vi "TestCloneAPI.vi"() -> ()   [LabVIEW 2018, in "SpecAnModule.lvlib"]
uses:
  SpecAnModule.lvlib
  TestInfo.ctl
  <userlib>/NIST/ModuleAdminLib/CloneRegistration/CloneRegistration.lvclass
  <userlib>/NIST/ModuleAdminLib/ModuleAdmin/ModuleAdmin.lvclass/ModuleAdmin.ctl
  <userlib>/NIST/ModuleAdminLib/ModuleAdmin/ModuleAdmin.lvclass
  PublicAPI/Arguments/Broadcasts/clDidInit.ctl
  PublicAPI/Arguments/Requests/clStopArgument.ctl
  SpecAnPlugins/SpecAnBaseClass/Typedefs/Waveform(s).ctl
  <userlib>/NIST/ModuleAdminLib/ModuleAdmin/Accessors/Read CloneRegRef.vi
  <userlib>/NIST/ModuleAdminLib/ModuleAdmin/Accessors/Write CloneRegRef.vi
  SpecAnPlugins/SpecAnBaseClass/SpecAnBase.lvclass
panel:
  out "Actual Points":i32[](array[numeric])
  out "Waveform Graph":T1(graph)
  in  "option string":string="Simulate=1,RangeCheck=1,QueryInstrStatus=0,Cache=1"
  in  "reset device (Yes)":bool=TRUE
  in  "id query (Yes)":bool=TRUE
  in  "btnAcqMode":bool
  out "TraceNames":string[](array[string])
  in  "btnInitiate":bool
  in  "btnGetTraceName":bool
  in  "btnConfigure":bool
  in  "btnAbortDevice":bool
  in  "btnCloseDevice":bool
  in  "btnInitDevice":bool
  in  "btnClear":bool
  in  "btnPref":bool
  in  "Show Panel":bool=TRUE
  in  "Plugin Type":u16(ring) items=["IVI Spectrum Analyzer"]
  in  "btnLoadPlugin":bool
  out "Path":path
  in  "btnRequestINIPath":bool
  in  "btnRemove":bool
  out "Status Log":string
  out "Active Modules (Array)":string[](array[string])
  in  "btnAdd":bool
  in  "btnStop":bool
  in  "Select Module":i32(ring)=-1 caption="Select Module to send Request" items=["All"=-1, "4140002"=4140002]
  # "Hidden"
  # "Visible"
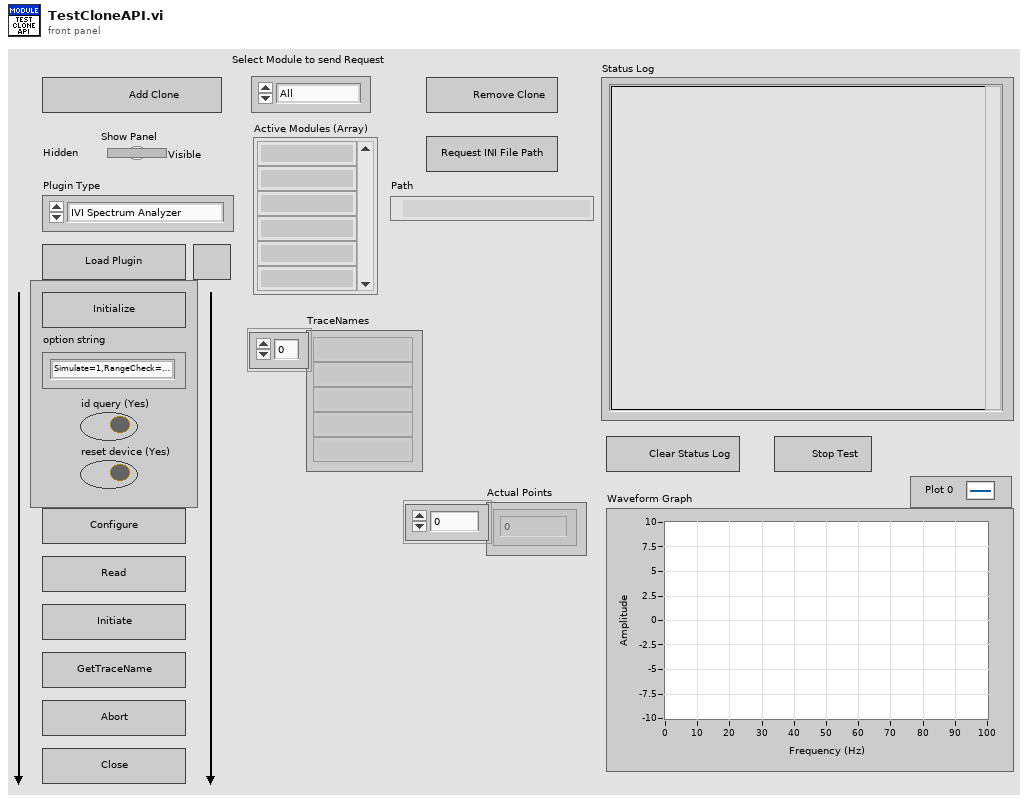
[diagram p1: front panel]
types:
  T1 = cluster{"Start Frequency (Hz)":dbl, "Delta Frequency(Hz)":dbl, "Amplitude":dbl[][]}
  T2 = typedef "SpecAnModule.lvlib/TestInfo.ctl" = cluster{"PluginIniFilePaths":path[]}
  T3 = cluster{"Status Log":refnum<vi>, "btnAdd":refnum<vi>, "btnStop":refnum<vi>, "Show Panel":refnum<vi>, "btnClear":refnum<vi>}
  T4 = typedef "SpecAnModule.lvlib/clBroadcastEvents.ctl" = cluster{"DidInit":refnum<user-event>, "StatusUpdate":refnum<user-event>, "ErrorReport":refnum<user-event>, "DidStop":refnum<user-event>, "PathToINI":refnum<user-event>, "TraceName":refnum<user-event>, "Reload Configuration File(s)":refnum<user-event>, "Measurements":refnum<user-event>}
  T5 = enum8{"Enabled", "Disabled", "Disabled and Grayed Out"}
  T6 = typedef "SpecAnModule.lvlib/clDidInit.ctl" = cluster{"Init?":bool, "ModuleAdmin":refnum<class "ModuleAdmin.lvclass">}
  T7 = typedef "SpecAnModule.lvlib/clStopArgument.ctl" = cluster{"Exit via Stop Module Req?":bool, "Wait for Module to stop?":bool, "ModuleAdmin":refnum<class "ModuleAdmin.lvclass">}
  T8 = typedef "SpecAnPlugins.lvlib/SpecAnBase.lvclass/Waveform(s).ctl" = cluster{"Actual Points":i32[], "Waveform Data":cluster{"Start Frequency (Hz)":dbl, "Delta Frequency(Hz)":dbl, "Amplitude":dbl[][]}}
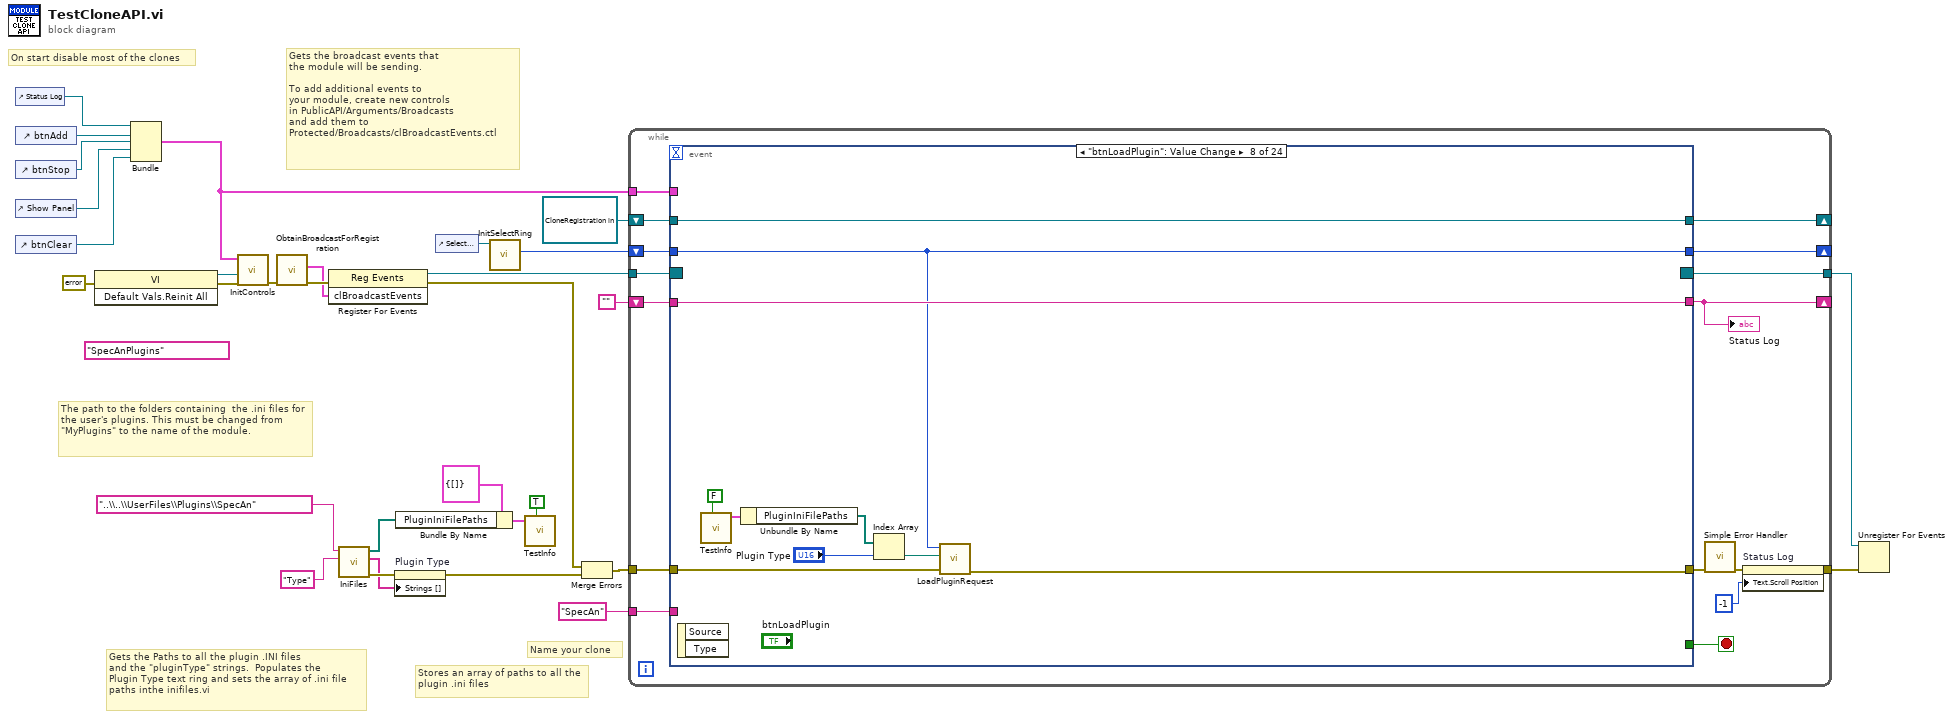
[diagram p0: block diagram]
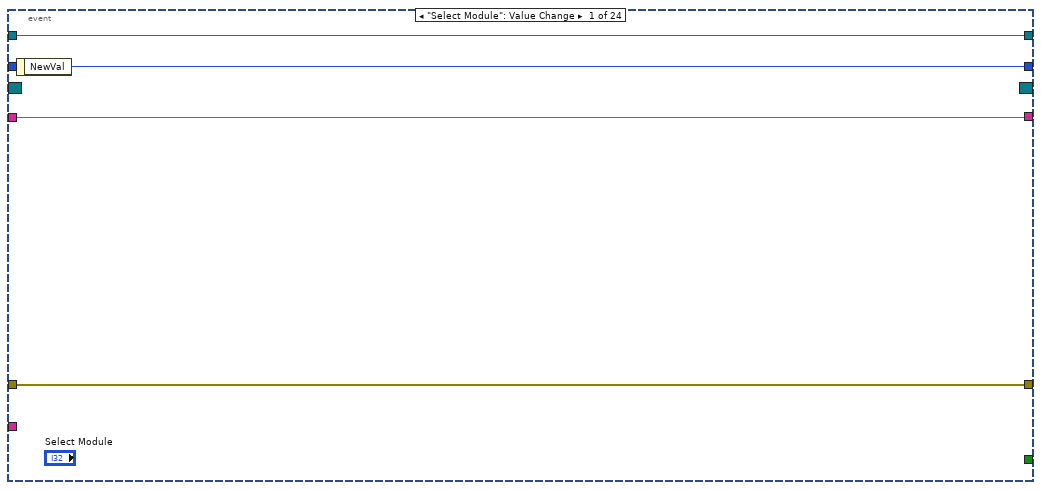
[diagram p2: hidden frame]
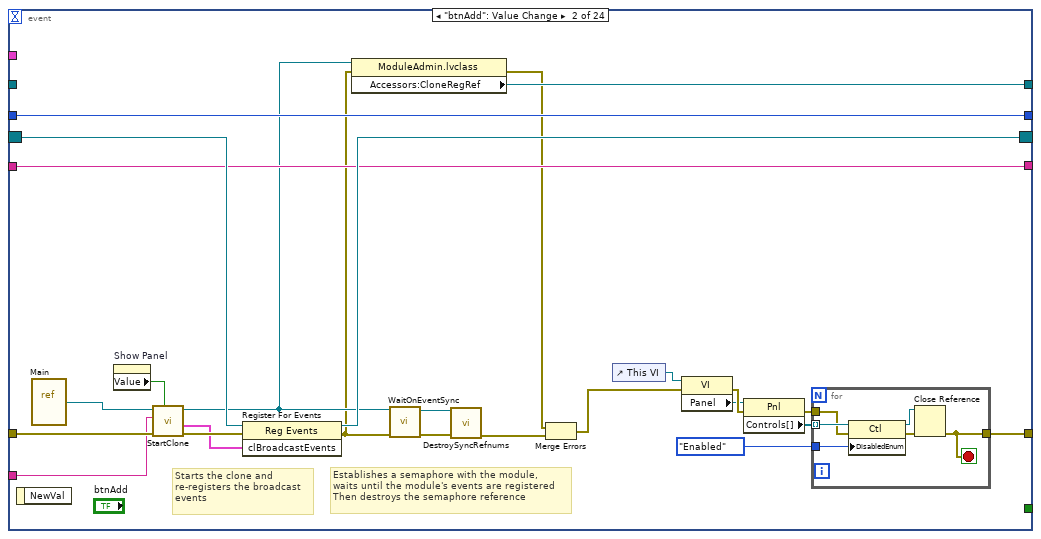
[diagram p3: hidden frame]
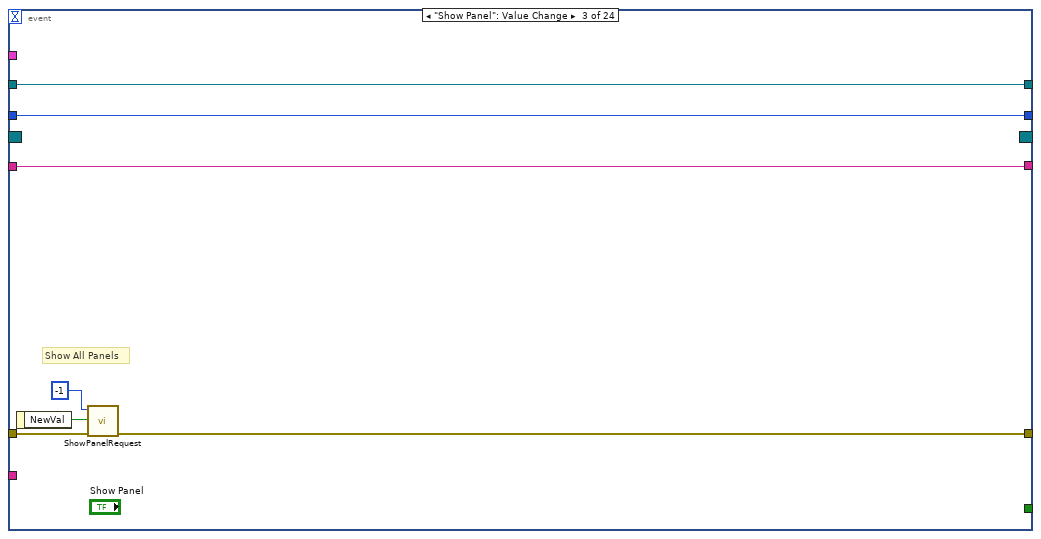
[diagram p4: hidden frame]
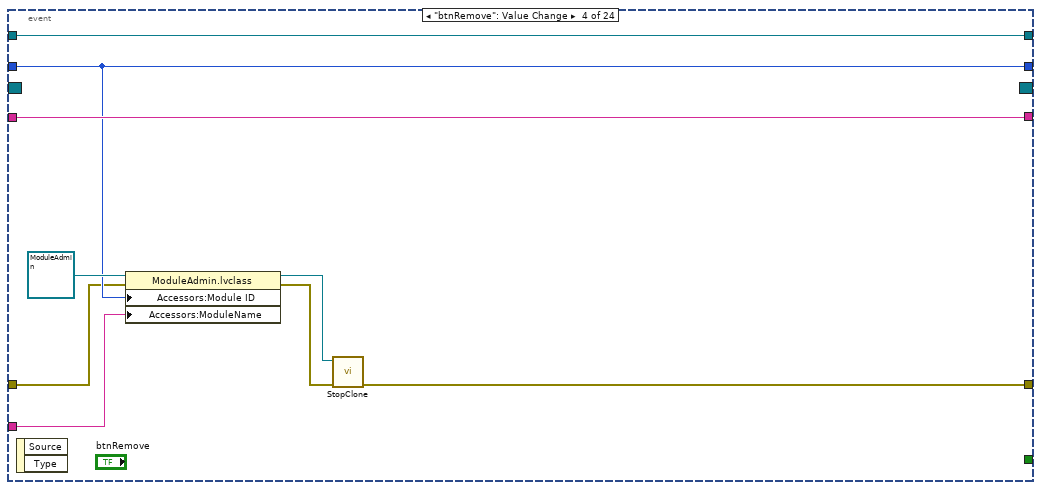
[diagram p5: hidden frame]
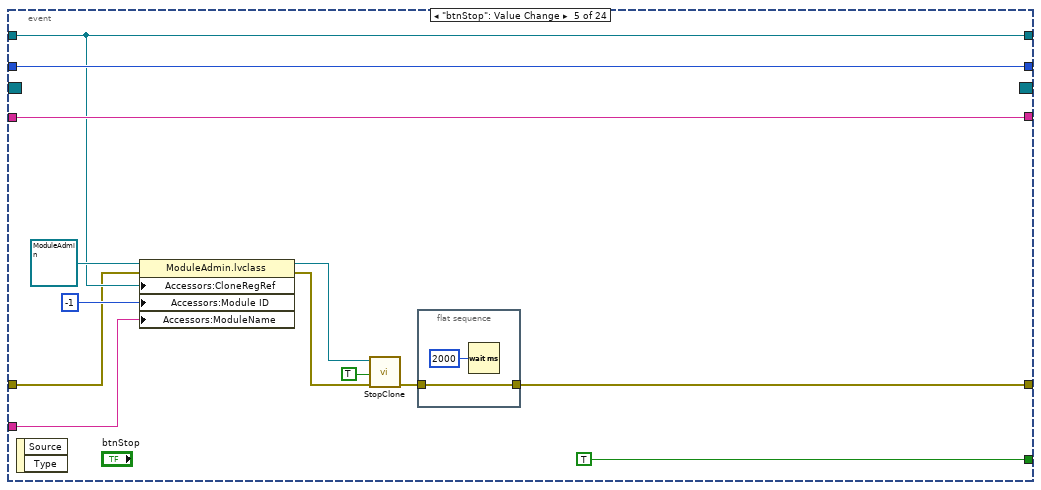
[diagram p6: hidden frame]
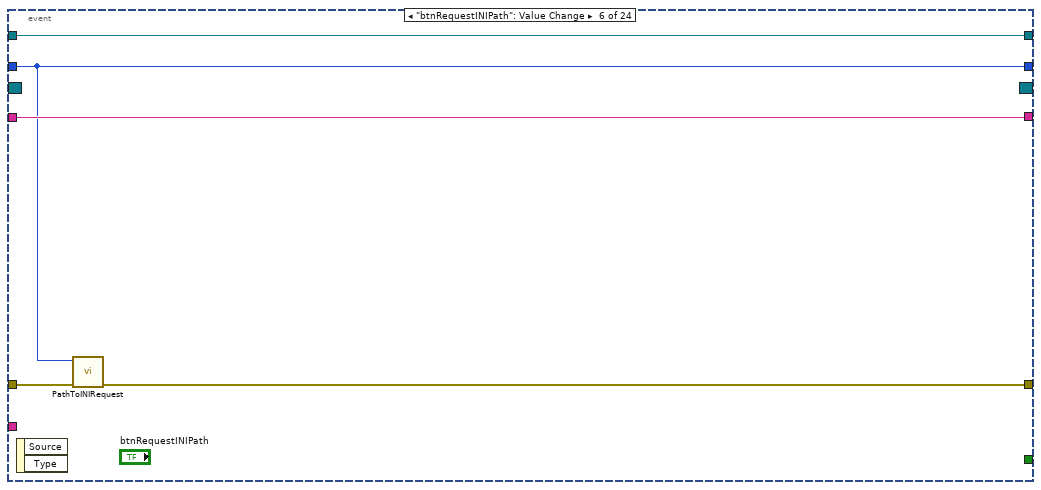
[diagram p7: hidden frame]
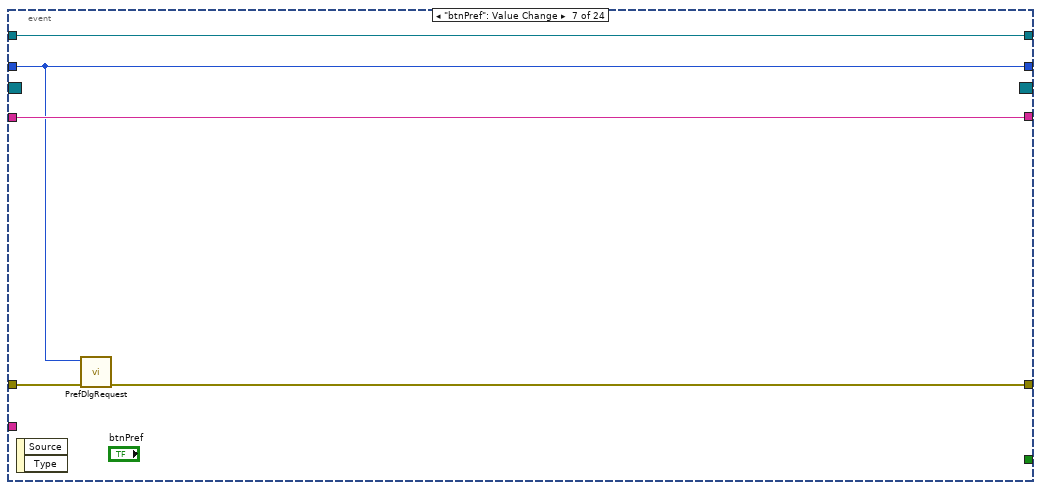
[diagram p8: hidden frame]
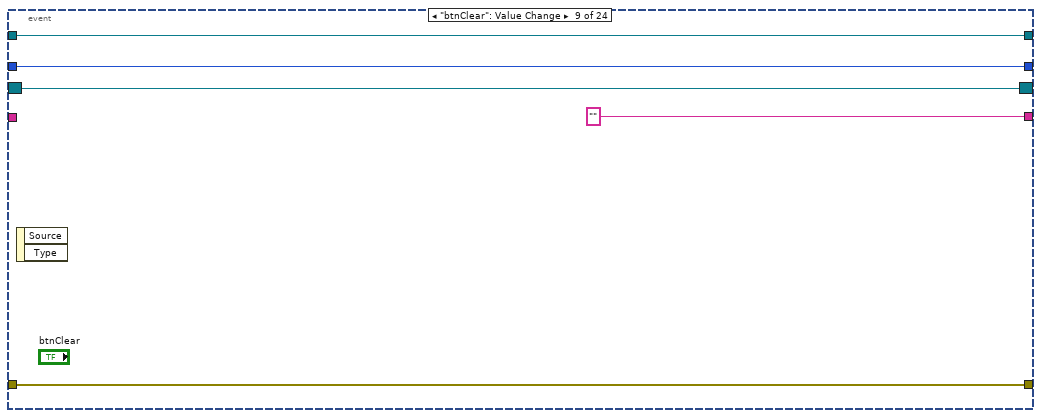
[diagram p9: hidden frame]
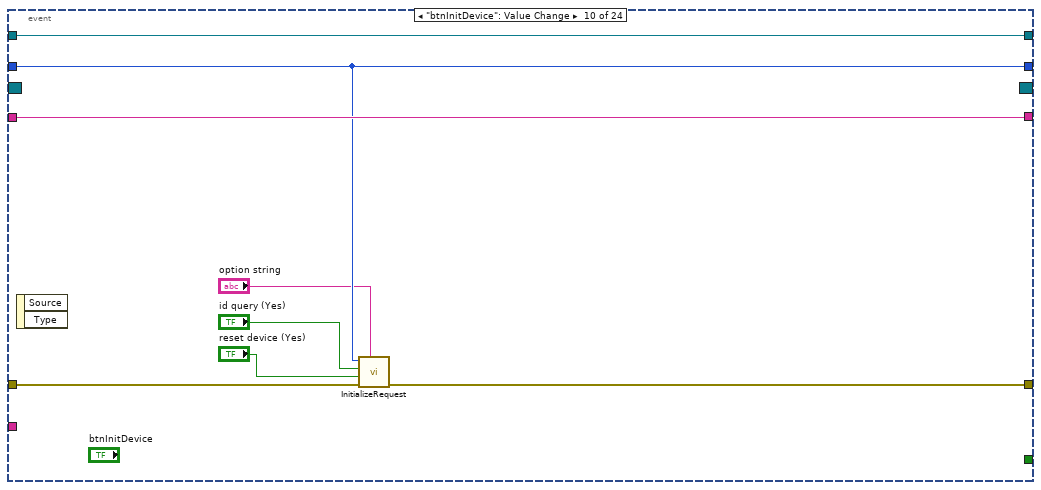
[diagram p10: hidden frame]
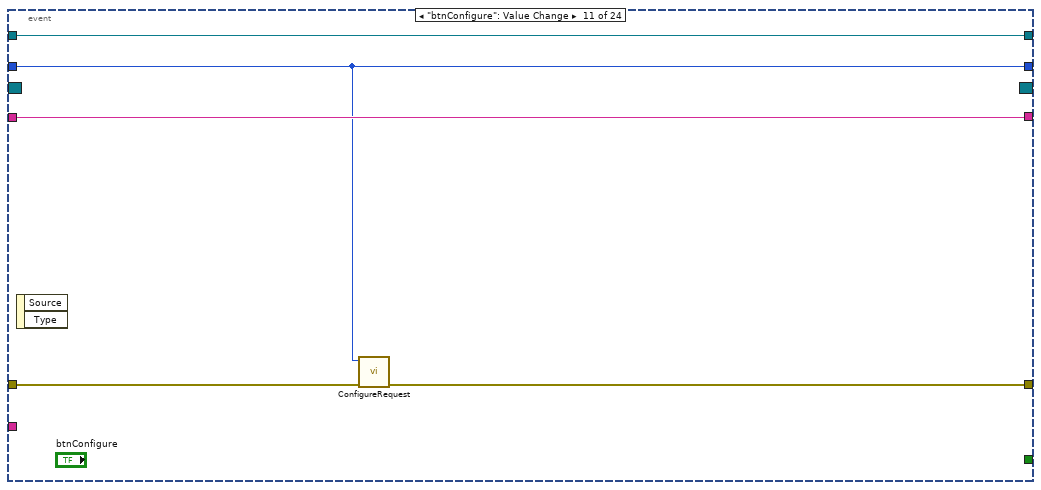
[diagram p11: hidden frame]
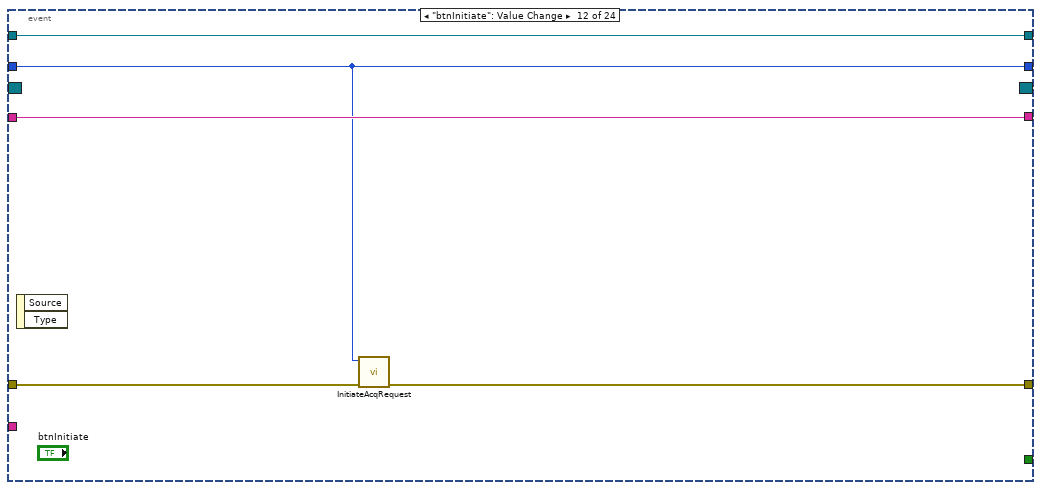
[diagram p12: hidden frame]
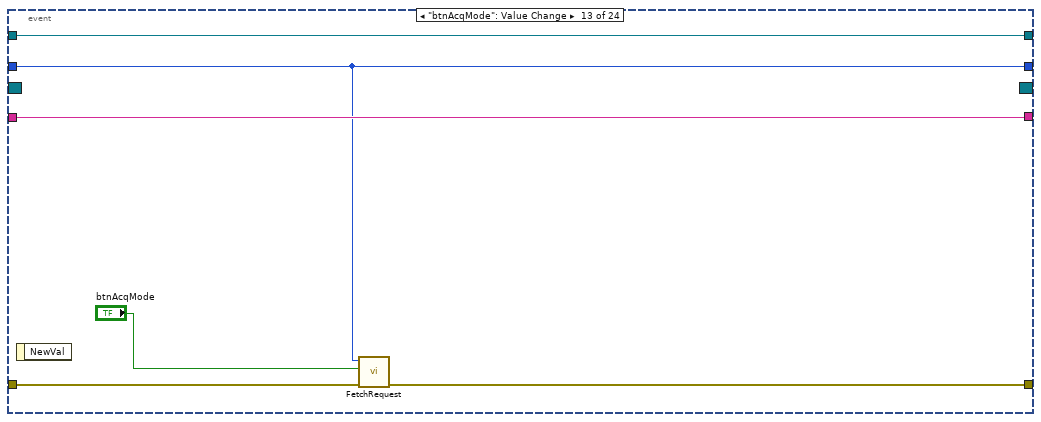
[diagram p13: hidden frame]
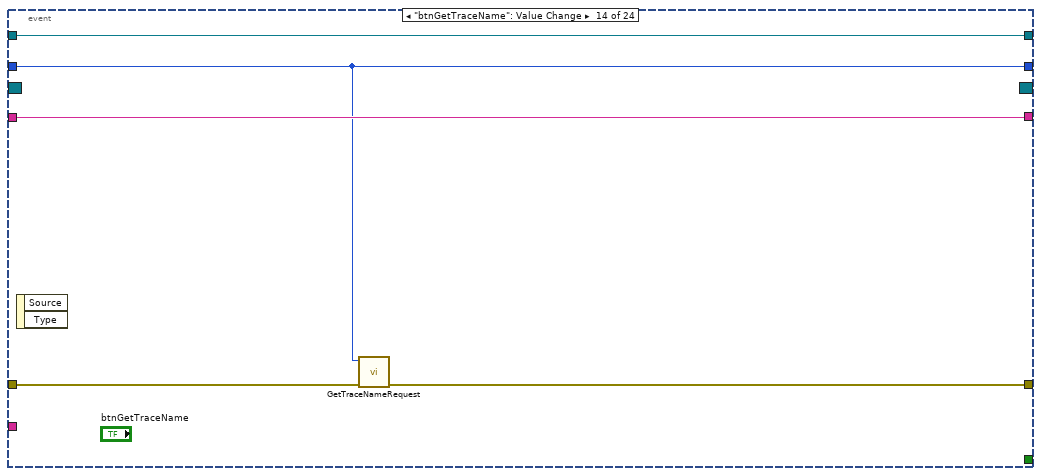
[diagram p14: hidden frame]
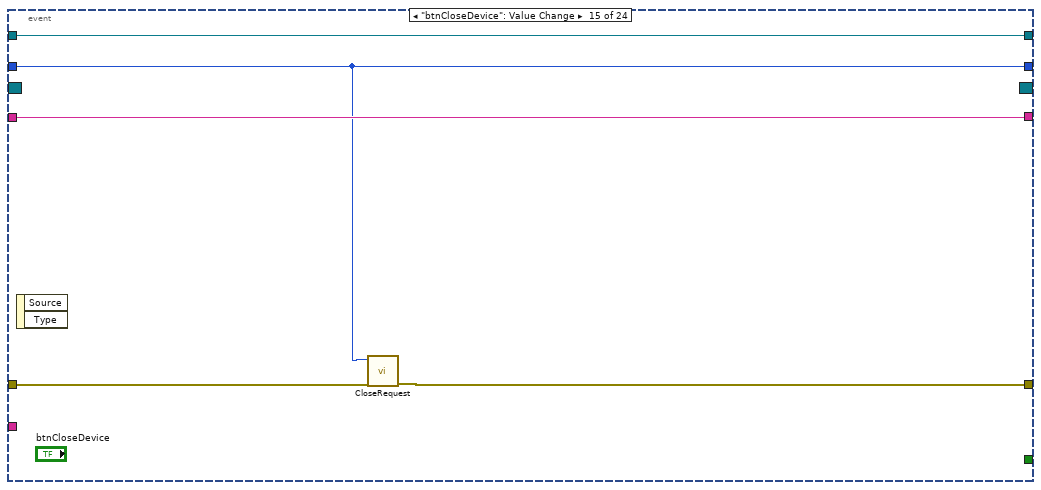
[diagram p15: hidden frame]
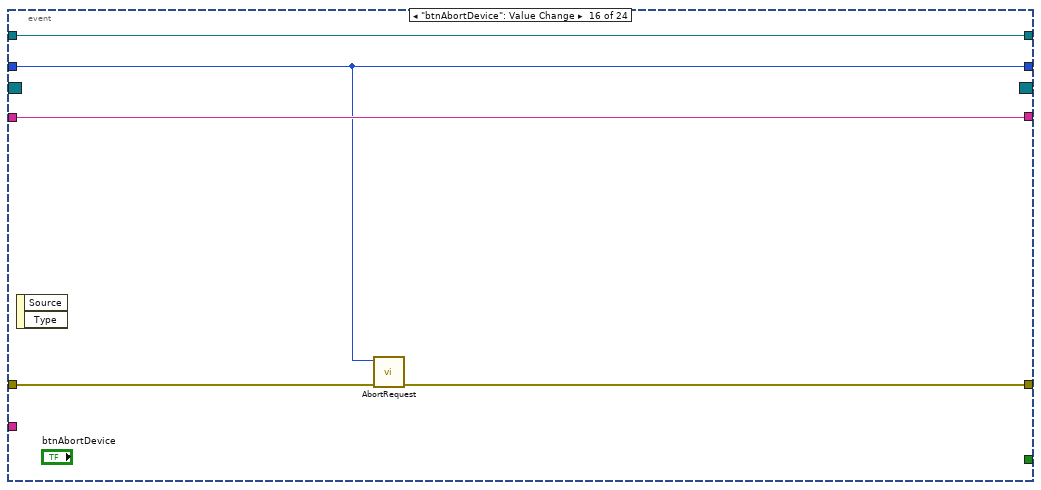
[diagram p16: hidden frame]
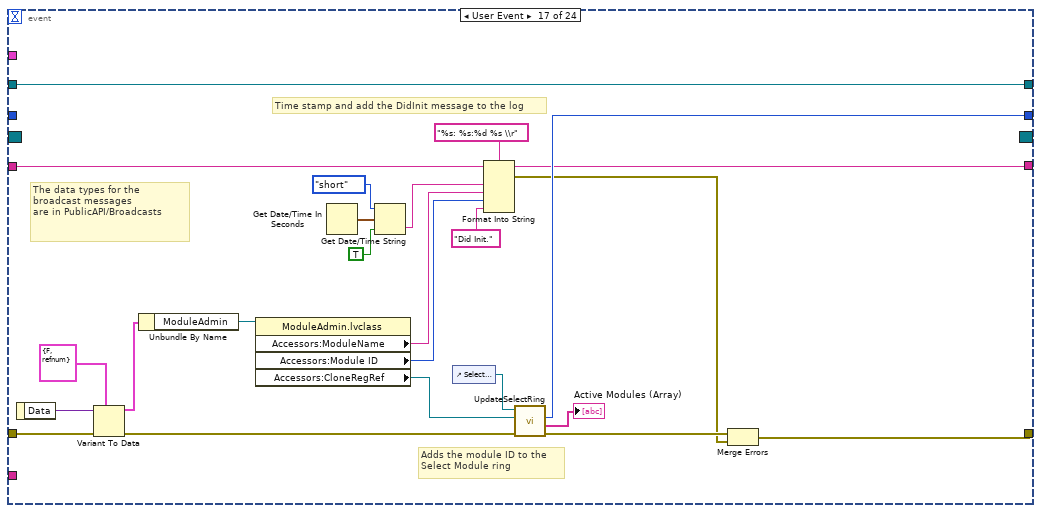
[diagram p17: hidden frame]
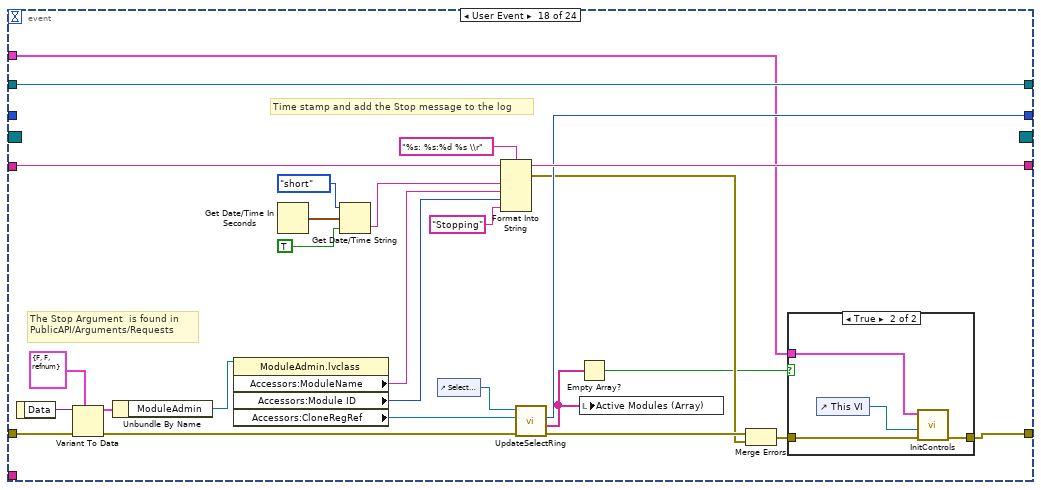
[diagram p18: hidden frame]
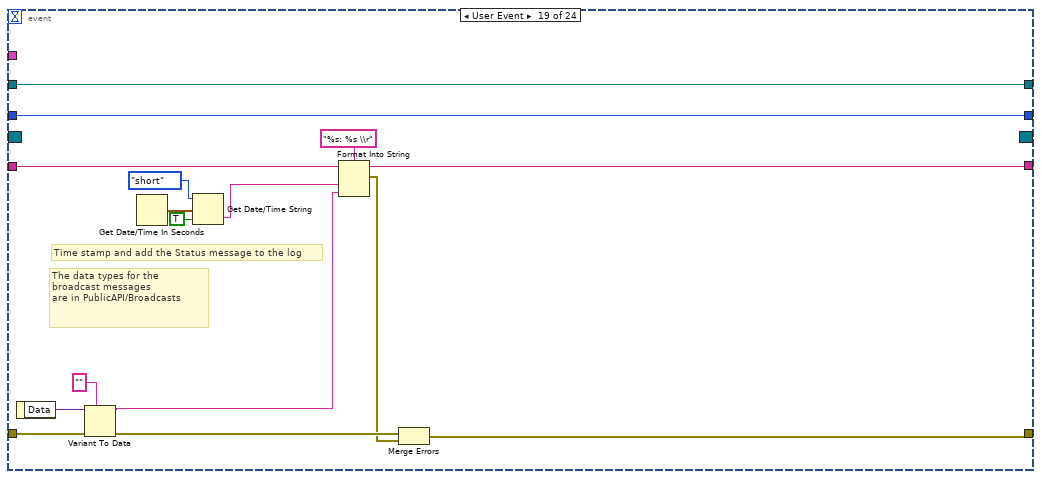
[diagram p20: hidden frame]
diagram:
  (unwired) "SpecAnPlugins" ("name or relative path")
  # "On start disable most of the clones"
  # "The path to the folders containing  the .ini files for the user's plugins. This must be changed from \"MyPlugins\" to the name of the module."
  # "Stores an array of paths to all the plugin .ini files"
  # "Gets the Paths to all the plugin .INI files\nand the \"pluginType\" strings.  Populates the \nPlugin Type text ring and sets the array of .ini file\npaths inthe inifiles.vi"
  # "Name your clone"
  # "Gets the broadcast events that\nthe module will be sending.\n\nTo add additional events to\nyour module, create new controls\nin PublicAPI/Arguments/Broadcasts\nand add them to\nProtected/Broadcasts/clBroadcastEvents.ctl"
  n1 = control-ref of="Status Log"() -> (w7:refnum<vi>)
  n2 = control-ref of="btnAdd"() -> (w6:refnum<vi>)
  n3 = control-ref of="btnStop"() -> (w5:refnum<vi>)
  n4 = control-ref of="Show Panel"() -> (w4:refnum<vi>)
  n5 = control-ref of="btnClear"() -> (w3:refnum<vi>)
  n6 = invoke class="VI" method="Default Vals.Reinit All"(error in=errorcluster {"status"=FALSE, "code"=0, "source"=""} ("error in (no error)")) -> (reference out=w11:refnum<vi>, error out=w10:errorcluster)  [unwired: 2 in, 1 out]
  n7 = Bundle("Status Log"=w7, "btnAdd"=w6, "btnStop"=w5, "Show Panel"=w4, "btnClear"=w3) -> (w2:T3)  [unwired: 1 in]
  n8 = call "InitControls.vi"("error in (no error)"=w10, "TestCloneAPI Reference"=w11, "Controls To Enable"=w2) -> ("error out"=w9:errorcluster)  [unwired: 8 in]
  n9 = call "ObtainBroadcastForRegistration.vi"("error in (no error)"=w9) -> ("error out"=w29:errorcluster, "clBroadcastEvents"=w28:T4)  [unwired: 9 in]
  n10 = register-events(error in=w29, w28) -> (reference out=w26:refnum<event-registration>, error out=w27:errorcluster)  [unwired: 1 in]
  n11 = call "IniFiles.vi"("iniKey"="Type", "name or relative path"="..\\..\\UserFiles\\Plugins\\SpecAn") -> ("error out"=w23:errorcluster, "Types"=w22:string[], "IniFilePaths"=w21:path[])  [unwired: 7 in]
  n12 = property on="Plugin Type" class="Ring (strict)"(error in=w23, "Strings []"=w22) -> (error out=w17:errorcluster)  [unwired: 1 in, 1 out]
  n13 = Bundle By Name(cluster=T2 {"PluginIniFilePaths"=[]} ("TestInfo"), "PluginIniFilePaths"=w21) -> (w20:T2)
  n14 = control-ref of="Select Module"() -> (w31:refnum<vi>)
  n15 = call "InitSelectRing.vi"("Ring Refnum"=w31) -> ("Module Ring Value"=w30:i32)  [unwired: 9 in, 1 out]
  n16 = call "TestInfo.vi"("Set (f)"=TRUE, "TestInfo 2"=w20) -> ()  [unwired: 9 in, 1 out]
  n17 = Merge Errors(w27, w17) -> (w18:errorcluster)
  n18 = while {
    shift-right: [w46] -> _
    shift-left: w30 -> [w47]
    tunnel: w18 -> [w44]
    tunnel: w26 -> [w42]
    tunnel: [w33] -> w14
    shift-right: [w41] -> _
    shift-left: "" -> [w40]
    tunnel: "SpecAn" ("ModuleName") -> [w39]
    tunnel: [w38] -> w13
    shift-right: [w37] -> _
    shift-left: refnum<data-value> refnum ("Accessors:CloneRegRef") -> [w36]
    tunnel: w2 -> [w32]
    stop <- w45 stop-if-true
    n19 = event shown="[7] \"btnLoadPlugin\": Value Change" {
      selector: w42 -> [_ w69 _ _ _ _ _ _ w136 _ _ _ _ _ _ _ _ _ _ _ _ _ _ _]
      dyn-events: [_ w68 _ _ _ _ _ _ w136 _ _ _ _ _ _ _ _ _ _ _ _ _ _ _] -> w38
      timeout: _ -> [_ _ _ _ _ _ _ _ _ _ _ _ _ _ _ _ _ _ _ _ _ _ _ _]
      tunnel: w47 -> [_ w76 w85 w93 w111 w117 w122 w130 w135 w143 w148 w153 w159 w164 w168 w173 _ _ w249 w253 w266 w272 w296 w307]
      tunnel: [w51 w76 w85 w93 w111 w117 w122 w130 w135 w143 w148 w153 w159 w164 w168 w173 w196 w216 w249 w253 w266 w272 w296 w307] -> w46
      tunnel: [_ _ _ _ TRUE _ _ _ _ _ _ _ _ _ _ _ _ _ _ _ _ FALSE _ FALSE] -> w45
      tunnel: w44 -> [w49 w75 w88 w91 w99 w116 w121 w132 w138 w145 w150 w155 w161 w166 w170 w174 w201 w224 w246 w258 w262 w276 w287 w314]
      tunnel: [w49 w58 w86 w92 w101 w115 w120 w131 w138 w142 w147 w152 w158 w163 w169 w175 w185 w204 w239 w257 w261 w269 w278 w299] -> w43
      tunnel: [w50 w66 w84 w98 w108 w118 w123 w133 "" w146 w151 w156 w162 w167 w172 w177 w189 w221 w242 w252 w267 w271 w279 w301] -> w41
      tunnel: w40 -> [w50 w66 w84 w98 w108 w118 w123 w133 _ w146 w151 w156 w162 w167 w172 w177 w188 w222 w248 w252 w267 w271 w281 w302]
      tunnel: w39 -> [_ w65 _ w96 w106 _ _ _ _ _ _ _ _ _ _ _ _ _ _ _ _ _ _ _]
      tunnel: [w48 w62 w83 w94 w103 w114 w119 w124 w134 w144 w149 w154 w160 w165 w171 w176 w178 w207 w234 w250 w260 w270 w297 _] -> w37
      tunnel: w36 -> [w48 _ w83 w94 w103 w114 w119 w124 w134 w144 w149 w154 w160 w165 w171 w176 w178 w207 w234 w250 w260 w270 w297 _]
      tunnel: w32 -> [_ _ _ _ _ _ _ _ _ _ _ _ _ _ _ _ _ w202 _ _ _ _ _ _]
      event "Select Module": Value Change {
        n20 = event-data() -> ("NewVal"=w51:i32)  [unwired: 1 in]
      }
      event "btnAdd": Value Change {
        # "Establishes a semaphore with the module,\nwaits until the module's events are registered\nThen destroys the semaphore reference"
        # "Starts the clone and\nre-registers the broadcast \nevents"
        n21 = event-data() -> ()  [unwired: 1 in, 1 out]
        n22 = vi-ref "Main.vi"() -> (w67:refnum<vi>)
        n23 = property on="Show Panel" class="Bool (strict)"() -> ("Value"=w64:bool)  [unwired: 2 in, 2 out]
        n24 = call "StartClone.vi"("ShowPanel? (f)"=w64, "error in (no error)"=w75, "ModuleName"=w65, "VI Refnum"=w67) -> ("error out"=w74:errorcluster, "clBroadcastEvents"=w71:T4, "ModuleAdmin"=w63:refnum<class "ModuleAdmin.lvclass">)  [unwired: 5 in]
        n25 = register-events(reference=w69, error in=w74, w71) -> (reference out=w68:refnum<event-registration>, error out=w61:errorcluster)
        n26 = property class="ModuleAdmin.lvclass"(reference=w63, error in=w61) -> (error out=w60:errorcluster, "Accessors:CloneRegRef"=w62:refnum<data-value>)  [unwired: 1 out]
        n27 = call <userlib>:"WaitOnEventSync.vi"("error in (no error)"=w61, "ModuleAdmin"=w63) -> ("error out"=w73:errorcluster, "ModuleAdmin"=w72:refnum<class "ModuleAdmin.lvclass">)  [unwired: 8 in]
        n28 = call <userlib>:"DestroySyncRefnums.vi"("error in (no error)"=w73, "ModuleAdmin"=w72) -> ("error out"=w70:errorcluster)  [unwired: 9 in]
        n29 = Merge Errors(w60, w70) -> (w59:errorcluster)
        n30 = control-ref of="This VI"() -> (w52:refnum<vi>)
        n31 = property class="VI"(reference=w52, error in=w59) -> (error out=w55:errorcluster, "Panel"=w53:refnum<vi>)  [unwired: 1 out]
        n32 = property class="Pnl"(reference=w53, error in=w55) -> (error out=w56:errorcluster, "Controls[]"=w54:refnum<vi>[])  [unwired: 1 out]
        n33 = for {
          tunnel: w54 -> [w82] mode=indexing
          tunnel: w56 -> [w81]
          tunnel: [w78] -> w58
          tunnel: T5."Enabled" ("Disabled") -> [w77]
          stop <- w78 stop-if-true
          n34 = property class="Ctl"(reference=w82, error in=w81, "DisabledEnum"=w77) -> (reference out=w79:refnum<vi>, error out=w80:errorcluster)
          n35 = Close Reference(reference=w79, error in (no error)=w80) -> (error out=w78:errorcluster)
        }
      }
      event "Show Panel": Value Change {
        # "Show All Panels"
        n36 = event-data() -> ("NewVal"=w89:bool)  [unwired: 1 in]
        n37 = call "ShowPanelRequest.vi"("error in (no error)"=w88, "ShowPanel?"=w89, "ModuleID"=-1) -> ("error out"=w86:errorcluster)  [unwired: 8 in]
      }
      event "btnRemove": Value Change {
        n38 = event-data() -> ()  [unwired: 1 in, 2 out]
        n39 = property class="ModuleAdmin.lvclass"(reference=refnum<class "ModuleAdmin.lvclass"> refnum ("ModuleAdmin.lvlib:ModuleAdmin.lvclass"), error in=w91, "Accessors:Module ID"=w93, "Accessors:ModuleName"=w96) -> (reference out=w95:refnum<class "ModuleAdmin.lvclass">, error out=w90:errorcluster)
        n40 = call "StopClone.vi"("error in (no error)"=w90, "ModuleAdmin"=w95) -> ("error out"=w92:errorcluster)  [unwired: 9 in]
      }
      event "btnStop": Value Change {
        n41 = event-data() -> ()  [unwired: 1 in, 2 out]
        n42 = property class="ModuleAdmin.lvclass"(reference=refnum<class "ModuleAdmin.lvclass"> refnum ("ModuleAdmin.lvlib:ModuleAdmin.lvclass"), error in=w99, "Accessors:CloneRegRef"=w103, "Accessors:Module ID"=-1 ("Module ID"), "Accessors:ModuleName"=w106) -> (reference out=w105:refnum<class "ModuleAdmin.lvclass">, error out=w100:errorcluster)
        n43 = call "StopClone.vi"("error in (no error)"=w100, "Wait for Module to stop?"=TRUE, "ModuleAdmin"=w105) -> ("error out"=w102:errorcluster)  [unwired: 8 in]
        n44 = flat-sequence {
          tunnel: w102 -> [w112]
          tunnel: [w112] -> w101
          frame #0 {
            n45 = Wait (ms)(milliseconds to wait=u32 2000) -> ()  [unwired: 1 out]
          }
        }
      }
      event "btnRequestINIPath": Value Change {
        n46 = event-data() -> ()  [unwired: 1 in, 2 out]
        n47 = call "PathToINIRequest.vi"("error in (no error)"=w116, "ModuleID"=w117) -> ("error out"=w115:errorcluster)  [unwired: 9 in]
      }
      event "btnPref": Value Change {
        n48 = event-data() -> ()  [unwired: 1 in, 2 out]
        n49 = call "PrefDlgRequest.vi"("error in (no error)"=w121, "ModuleID"=w122) -> ("error out"=w120:errorcluster)  [unwired: 9 in]
      }
      event "btnLoadPlugin": Value Change {
        n50 = event-data() -> ()  [unwired: 1 in, 2 out]
        n51 = call "TestInfo.vi"("Set (f)"=FALSE) -> ("TestInfo"=w128:T2)  [unwired: 10 in]
        n52 = Unbundle By Name(w128) -> ("PluginIniFilePaths"=w127:path[])
        n53 = Index Array(array=w127, index="Plugin Type") -> (element=w125:path)
        n54 = call "LoadPluginRequest.vi"("error in (no error)"=w132, "PathToPluginINI"=w125, "ModuleID"=w130) -> ("error out"=w131:errorcluster)  [unwired: 8 in]
      }
      event "btnClear": Value Change {
        n55 = event-data() -> ()  [unwired: 1 in, 2 out]
      }
      event "btnInitDevice": Value Change {
        n56 = event-data() -> ()  [unwired: 1 in, 2 out]
        n57 = call "InitializeRequest.vi"("option string"="option string", "error in (no error)"=w145, "reset device (Yes)"="reset device (Yes)", "id query (Yes)"="id query (Yes)", "ModuleID"=w143) -> ("error out"=w142:errorcluster)  [unwired: 6 in]
      }
      event "btnConfigure": Value Change {
        n58 = event-data() -> ()  [unwired: 1 in, 2 out]
        n59 = call "ConfigureRequest.vi"("error in (no error)"=w150, "ModuleID"=w148) -> ("error out"=w147:errorcluster)  [unwired: 9 in]
      }
      event "btnInitiate": Value Change {
        n60 = event-data() -> ()  [unwired: 1 in, 2 out]
        n61 = call "InitiateAcqRequest.vi"("error in (no error)"=w155, "ModuleID"=w153) -> ("error out"=w152:errorcluster)  [unwired: 9 in]
      }
      event "btnAcqMode": Value Change {
        n62 = event-data() -> ()  [unwired: 1 in, 1 out]
        n63 = call "FetchRequest.vi"("error in (no error)"=w161, "AcqMode"="btnAcqMode", "ModuleID"=w159) -> ("error out"=w158:errorcluster)  [unwired: 8 in]
      }
      event "btnGetTraceName": Value Change {
        n64 = event-data() -> ()  [unwired: 1 in, 2 out]
        n65 = call "GetTraceNameRequest.vi"("error in (no error)"=w166, "ModuleID"=w164) -> ("error out"=w163:errorcluster)  [unwired: 9 in]
      }
      event "btnCloseDevice": Value Change {
        n66 = event-data() -> ()  [unwired: 1 in, 2 out]
        n67 = call "CloseRequest.vi"("error in (no error)"=w170, "ModuleID"=w168) -> ("error out"=w169:errorcluster)  [unwired: 9 in]
      }
      event "btnAbortDevice": Value Change {
        n68 = event-data() -> ()  [unwired: 1 in, 2 out]
        n69 = call "AbortRequest.vi"("error in (no error)"=w174, "ModuleID"=w173) -> ("error out"=w175:errorcluster)  [unwired: 9 in]
      }
      event User Event {
        # "Adds the module ID to the \nSelect Module ring"
        # "Time stamp and add the DidInit message to the log"
        # "The data types for the broadcast messages\nare in PublicAPI/Broadcasts"
        n70 = event-data() -> ("Data"=w200:variant)  [unwired: 1 in]
        n71 = Variant To Data(error in=w201, type=T6 {"Init?"=FALSE, "ModuleAdmin"=refnum} ("clDidInit"), Variant=w200) -> (data=w193:T6, error out=w198:errorcluster)
        n72 = Unbundle By Name(w193) -> ("ModuleAdmin"=w183:refnum<class "ModuleAdmin.lvclass">)
        n73 = property class="ModuleAdmin.lvclass"(reference=w183) -> ("Accessors:ModuleName"=w181:string, "Accessors:Module ID"=w180:i32, "Accessors:CloneRegRef"=w179:refnum<data-value>)  [unwired: 1 in, 2 out]
        n74 = Get Date/Time In Seconds() -> (seconds since 1Jan1904=w191:timestamp)
        n75 = Get Date/Time String(date format (0)=enum16{"short", "long", "abbreviated"}."short", seconds (now)=w191, want seconds? (F)=TRUE) -> (time string=w194:string)  [unwired: 1 out]
        n76 = control-ref of="Select Module"() -> (w197:refnum<vi>)
        n77 = Format Into String(format string="%s: %s:%d %s \\r", initial string=w188, w194, w181, w180, "Did Init.") -> (resulting string=w189:string, error out=w186:errorcluster)  [unwired: 1 in]
        n78 = call "UpdateSelectRing.vi"("error in (no error)"=w198, "CloneRegRef"=w179, "Ring Refnum"=w197) -> ("error out"=w187:errorcluster, "ActiveModules"=→"Active Modules (Array)":string[], "Module Ring Value"=w196:i32)  [unwired: 6 in]
        n79 = Merge Errors(w187, w186) -> (w185:errorcluster)
      }
      event User Event {
        # "Time stamp and add the Stop message to the log"
        # "The Stop Argument  is found in\nPublicAPI/Arguments/Requests"
        n80 = event-data() -> ("Data"=w223:variant)  [unwired: 1 in]
        n81 = Variant To Data(error in=w224, type=T7 {"Exit via Stop Module Req?"=FALSE, "Wait for Module to stop?"=FALSE, "ModuleAdmin"=refnum} ("Stop Argument"), Variant=w223) -> (data=w219:T7, error out=w218:errorcluster)
        n82 = Unbundle By Name(w219) -> ("ModuleAdmin"=w212:refnum<class "ModuleAdmin.lvclass">)
        n83 = property class="ModuleAdmin.lvclass"(reference=w212) -> ("Accessors:ModuleName"=w210:string, "Accessors:Module ID"=w209:i32, "Accessors:CloneRegRef"=w208:refnum<data-value>)  [unwired: 1 in, 2 out]
        n84 = Get Date/Time In Seconds() -> (seconds since 1Jan1904=w226:timestamp)
        n85 = Get Date/Time String(date format (0)=enum16{"short", "long", "abbreviated"}."short", seconds (now)=w226, want seconds? (F)=TRUE) -> (time string=w228:string)  [unwired: 1 out]
        n86 = control-ref of="Select Module"() -> (w217:refnum<vi>)
        n87 = Format Into String(format string="%s: %s:%d %s \\r", initial string=w222, w228, w210, w209, "Stopping") -> (resulting string=w221:string, error out=w214:errorcluster)  [unwired: 1 in]
        n88 = call "UpdateSelectRing.vi"("error in (no error)"=w218, "CloneRegRef"=w208, "Ring Refnum"=w217) -> ("error out"=w215:errorcluster, "ActiveModules"=w206:string[], "Module Ring Value"=w216:i32)  [unwired: 6 in]
        n89 = Empty Array?(array=w206) -> (empty?=w203:bool)
        n90 = local write "Active Modules (Array)"(w206) -> ()
        n91 = Merge Errors(w215, w214) -> (w205:errorcluster)
        n92 = case shown="True" w203 {
          tunnel: w205 -> [w229 w233]
          tunnel: [w229 w232] -> w204
          tunnel: w202 -> [_ w230]
          frame False {
          }
          frame True {
            n93 = control-ref of="This VI"() -> (w231:refnum<vi>)
            n94 = call "InitControls.vi"("error in (no error)"=w233, "TestCloneAPI Reference"=w231, "Controls To Enable"=w230) -> ("error out"=w232:errorcluster)  [unwired: 8 in]
          }
        }
      }
      event User Event {
        # "Time stamp and add the Status message to the log"
        # "The data types for the broadcast messages\nare in PublicAPI/Broadcasts"
        n95 = event-data() -> ("Data"=w245:variant)  [unwired: 1 in]
        n96 = Variant To Data(error in=w246, type="" ("clStatUpdate"), Variant=w245) -> (data=w235:string, error out=w241:errorcluster)
        n97 = Get Date/Time In Seconds() -> (seconds since 1Jan1904=w243:timestamp)
        n98 = Get Date/Time String(date format (0)=enum16{"short", "long", "abbreviated"}."short", seconds (now)=w243, want seconds? (F)=TRUE) -> (time string=w236:string)  [unwired: 1 out]
        n99 = Format Into String(format string="%s: %s \\r", initial string=w248, w236, w235) -> (resulting string=w242:string, error out=w240:errorcluster)  [unwired: 1 in]
        n100 = Merge Errors(w241, w240) -> (w239:errorcluster)
      }
      event User Event {
        # "#CodeNeeded\nThis is a very crude error handler\nA better error handler will be needed"
        # "The data types for the broadcast messages\nare in PublicAPI/Broadcasts"
        n101 = event-data() -> ("ModuleID"=w255:i32, "Data"=w259:variant)  [unwired: 1 in]
        n102 = Variant To Data(error in=w258, type=errorcluster {"status"=FALSE, "code"=0, "source"=""} ("Cluster"), Variant=w259) -> (data=w251:errorcluster, error out=w257:errorcluster)
        n103 = Number To Decimal String(number=w255) -> (decimal integer string=w254:string)  [unwired: 1 in]
        n104 = call <vilib>:"General Error Handler.vi"("[error source] (\" \")"=w254, "error in (no error)"=w251) -> ()  [unwired: 9 in, 5 out]
      }
      event User Event {
        n105 = event-data() -> ("Data"=w264:variant)  [unwired: 1 in, 1 out]
        n106 = Variant To Data(error in=w262, type=path "" ("Path"), Variant=w264) -> (data=→"Path":path, error out=w261:errorcluster)
      }
      event User Event {
        n107 = event-data() -> ("Data"=w275:variant)  [unwired: 1 in]
        n108 = Variant To Data(error in=w276, type=string[] [] ("Array"), Variant=w275) -> (data=→"TraceNames":string[], error out=w269:errorcluster)
      }
      event User Event {
        n109 = event-data() -> ()  [unwired: 1 in, 1 out]
        n110 = call "IniFiles.vi"("error in"=w287, "iniKey"="Type", "name or relative path"="..\\..\\UserFiles\\Plugins\\SpecAn") -> ("error out"=w288:errorcluster, "Types"=w289:string[], "IniFilePaths"=w290:path[])  [unwired: 6 in]
        n111 = property on="Plugin Type" class="Ring (strict)"(error in=w288, "Strings []"=w289) -> (error out=w280:errorcluster)  [unwired: 1 in, 1 out]
        n112 = Bundle By Name(cluster=T2 {"PluginIniFilePaths"=[]} ("TestInfo"), "PluginIniFilePaths"=w290) -> (w291:T2)
        n113 = Get Date/Time In Seconds() -> (seconds since 1Jan1904=w285:timestamp)
        n114 = call "TestInfo.vi"("Set (f)"=TRUE, "TestInfo 2"=w291) -> ()  [unwired: 9 in, 1 out]
        n115 = Get Date/Time String(date format (0)=enum16{"short", "long", "abbreviated"}."short", seconds (now)=w285, want seconds? (F)=TRUE) -> (time string=w286:string)  [unwired: 1 out]
        n116 = Format Into String(format string="%s: %s \\r", initial string=w281, error in=w280, w286, "INI File Reloaded") -> (resulting string=w279:string, error out=w278:errorcluster)
      }
      event User Event {
        (unwired) TRUE ("want seconds? (F)")
        n117 = event-data() -> ("Data"=w313:variant)  [unwired: 1 in]
        n118 = Variant To Data(error in=w314, type=T8 {"Actual Points"=[], "Waveform Data"={"Start Frequency (Hz)"=0.0, "Delta Frequency(Hz)"=0.0, "Amplitude"=[]}} ("Waveform(s)"), Variant=w313) -> (data=w310:T8, error out=w300:errorcluster)
        n119 = Unbundle By Name(w310) -> ("Actual Points"=→"Actual Points":i32[], "Waveform Data"=→"Waveform Graph":T1)
        n120 = Get Date/Time In Seconds() -> (seconds since 1Jan1904=w306:timestamp)
        n121 = Get Date/Time String(date format (0)=enum16{"short", "long", "abbreviated"}."short", seconds (now)=w306) -> (time string=w305:string)  [unwired: 1 in, 1 out]
        n122 = Format Into String(format string="%s: %s \\r", initial string=w302, error in=w300, w305, "MeasurementsTaken" ("input 2")) -> (resulting string=w301:string, error out=w299:errorcluster)
      }
    }
    "Status Log" <- w41
    n123 = call <vilib>:"Simple Error Handler.vi"("error in (no error)"=w43) -> ("error out"=w34:errorcluster)  [unwired: 4 in, 4 out]
    n124 = property on="Status Log" class="Str"(error in=w34, "Text.Scroll Position"=-1) -> (error out=w33:errorcluster)  [unwired: 1 in, 1 out]
  }
  n125 = Unregister For Events(event registration refnum=w13, error in=w14) -> ()  [unwired: 1 out]
